vi "Create.vi"(8 "error in (no error)":errorcluster, 11 "Event name":string) -> (0 "error out":errorcluster, 3 "Event out":refnum<class "Event.lvclass">)   [LabVIEW 2015, in "MDSplus.lvlib" / "Event.lvclass"]
uses:
  <vilib>/MDSplus/Classes/Event_Class/Event.lvclass
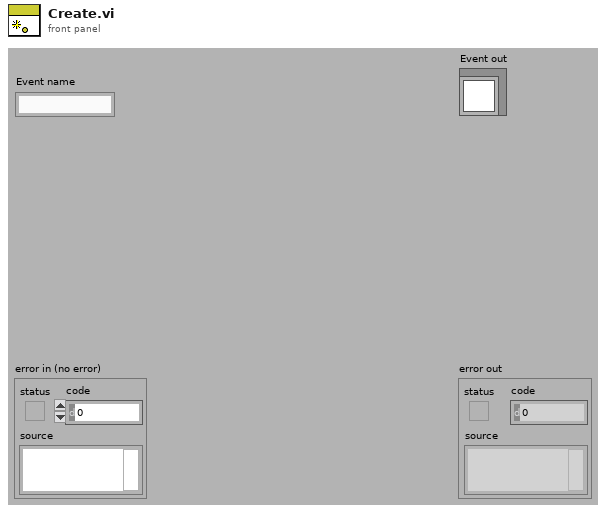
[diagram p1: front panel]
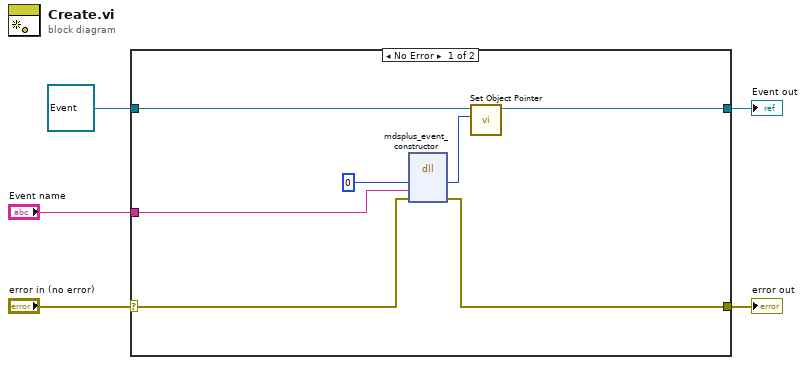
[diagram p0: block diagram]
diagram:
  n1 = case shown="No Error" "error in (no error)" {
    selector: "error in (no error)" -> [w7 w14]
    tunnel: [w6 w14] -> w4
    tunnel: [w9 w13] -> w2
    tunnel: refnum<class "Event.lvclass"> refnum ("Tree in") -> [w10 w13]
    tunnel: "Event name" -> [w11 _]
    frame No Error {
      n2 = dll-call lib="MDSobjectsLVShr" fn="mdsplus_event_constructor"("lvEventPtr"=i64 0 ("lvTreePtr"), "evNameIn"=w11, "error"=w7) -> ("lvEventPtr"=w8:i64, "error"=w6:errorcluster)  [unwired: 5 in, 2 out]
      n3 = call-dynamic "Set Object Pointer.vi"("Object Pointer"=w8, "Event in"=w10) -> ("Event out"=w9:refnum<class "Event.lvclass">)  [unwired: 9 in]
    }
    frame Error {
    }
  }
  "error out" <- w4
  "Event out" <- w2
